vi "Write ID.vi"(8 "error in":errorcluster, 10 "ID":string, 11 "Configurable Device in":refnum<class "Configurable Device.lvclass">) -> (0 "error out":errorcluster, 3 "Configurable Device out":refnum<class "Configurable Device.lvclass">)   [LabVIEW 2016, in "Configurable Device.lvclass"]
uses:
  Configurable Device.lvclass
  Configurable Device.lvclass/Configurable Device.ctl
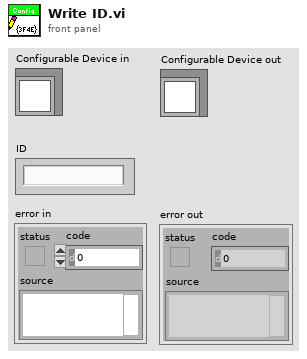
[diagram p1: front panel]
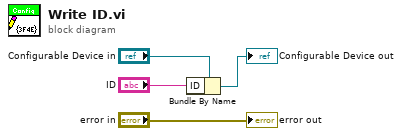
[diagram p0: block diagram]
diagram:
  n1 = Bundle By Name(cluster="Configurable Device in", "ID"="ID") -> (→"Configurable Device out":refnum<class "Configurable Device.lvclass">)
  "error out" <- "error in"
